vi "isDsc.vi"(8 "error in (no error)":errorcluster) -> (0 "error out":errorcluster, 2 "isDsc2":bool, 3 "isDsc1":bool)   [LabVIEW 2015, in "ESLSCDLL.lvlib"]
uses:
  ESLSCDLL.lvlib
  Globals.vi
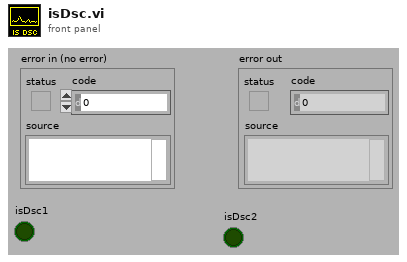
[diagram p1: front panel]
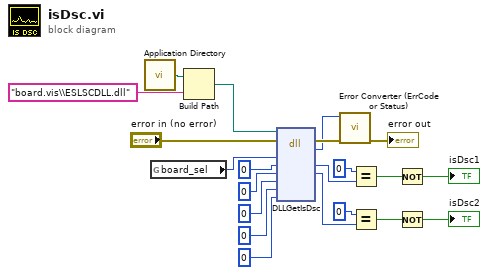
[diagram p0: block diagram]
diagram:
  n1 = call <vilib>:"Application Directory.vi"() -> ("Application Directory"=w11:path)
  n2 = global read "Globals.vi" "board_sel"() -> (w8:u32)
  n3 = Build Path(base path=w11, name or relative path="board.vis\\ESLSCDLL.dll") -> (appended path=w9:path)
  n4 = dll-call lib="C:/ENTW/PCIE/LV64/board.vis/ESLSCDLL.dll" fn="DLLGetIsDsc" ("lwlscdll.dll:DLLWriteLongS0")(path in=w9, error in="error in (no error)", "board_sel"=w8, "isDsc0"=u8 0, "isDsc1"=u8 0, "isDsc2"=u8 0, "isDsc3"=u8 0, "isDsc4"=u8 0) -> (error out=w13:errorcluster, "es_status_codes"=w12:i32, "isDsc0"=w2:u8, "isDsc1"=w1:u8)  [unwired: 5 in, 1 out]
  n5 = call "Error Converter (ErrCode or Status).vi"("error in (no error)"=w13, "error code"=w12) -> ("error out"=→"error out":errorcluster)  [unwired: 9 in]
  n6 = Equal?(x=u8 0, y=w2) -> (x = y?=w20:bool)
  n7 = Equal?(x=u8 0, y=w1) -> (x = y?=w17:bool)
  n8 = Not(x=w20) -> (.not. x?=→"isDsc1":bool)
  n9 = Not(x=w17) -> (.not. x?=→"isDsc2":bool)
